vi "RT Driver VI.vi"(6 "Device Clock":string, 9 "Device Inputs FIFO":refnum<k33>, 10 "Device Outputs FIFO":refnum<k33>, 11 "Device Reference":T1 format="%.0x") -> ()   [LabVIEW 2017, in "CD_CI_Test Engine.lvlib"]
uses:
  CD_CI_Test Engine.lvlib
  <vilib>/NI Veristand/Custom Device API/Custom Device Channel Type.ctl
  <vilib>/NI VeriStand/Custom Device API/Custom Device API.lvlib
  <vilib>/NI VeriStand/Custom Device Tools/Custom Device Utility Library/Custom Device Utility Library.lvlib
  <vilib>/NI Veristand/Custom Device API/Custom Device Item Ref.ctl
panel:
  in  "Initialization Status Notifier":refnum<notifier>
  in  "Status Notifier":refnum<notifier>
  # "Custom Device Template\nv1.0"
  # "Use this template as a starting point for creating a custom device code module. The input controls shown here are specially named controls that the system will use to provide the device loop with data. The controls are not required for the device loop to run. For instance, if the device doesn't produce any output data, then you don't need the Device Outputs FIFO control. If you do use these controls, however, they need to have these exact names to be functional."
  # "The optional status notifier element is used to notify the RT engine of the last state of the custom device, and to indicate the device has completed execution. If this control is not used, a default No Error value is returned to the system when the device finishes execution.\n\nNote: This error state is not checked until the system shuts down. Use an output status channel to send more immediate status values to the system."
  # "This optional input can be used to send the VeriStand Engine the final status of the custom device initalization process. If this control exists on the custom device front panel, the VeriStand Engine will wait for a status update before starting up. If the custom device reports an error, that will abort the execution of the current configuration in the VeriStand Engine.\n\nThis control can be deleted if the custom device does not need to send the initialization status update."
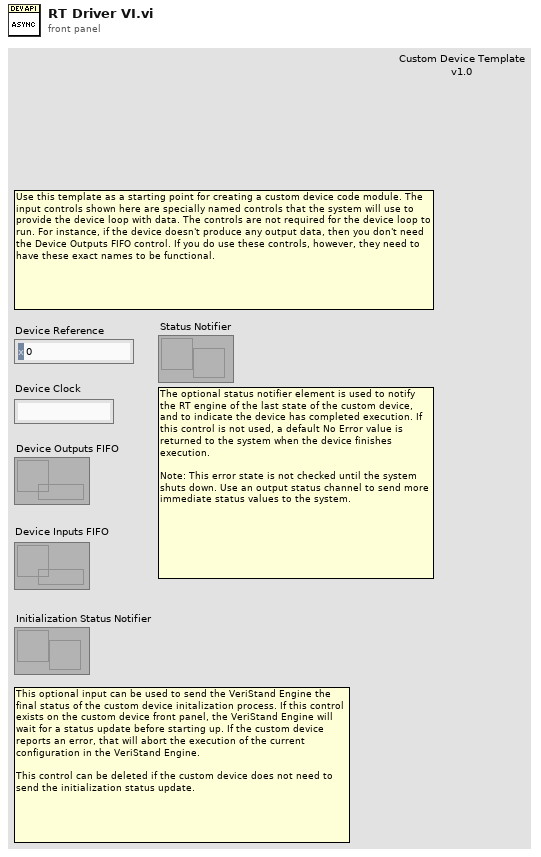
[diagram p1: front panel]
types:
  T1 = typedef "Custom Device API.lvlib/Custom Device Item Ref.ctl" = u64
  T2 = typedef "Custom Device API.lvlib/Custom Device Channel Type.ctl" = enum16{"Input", "Output"}
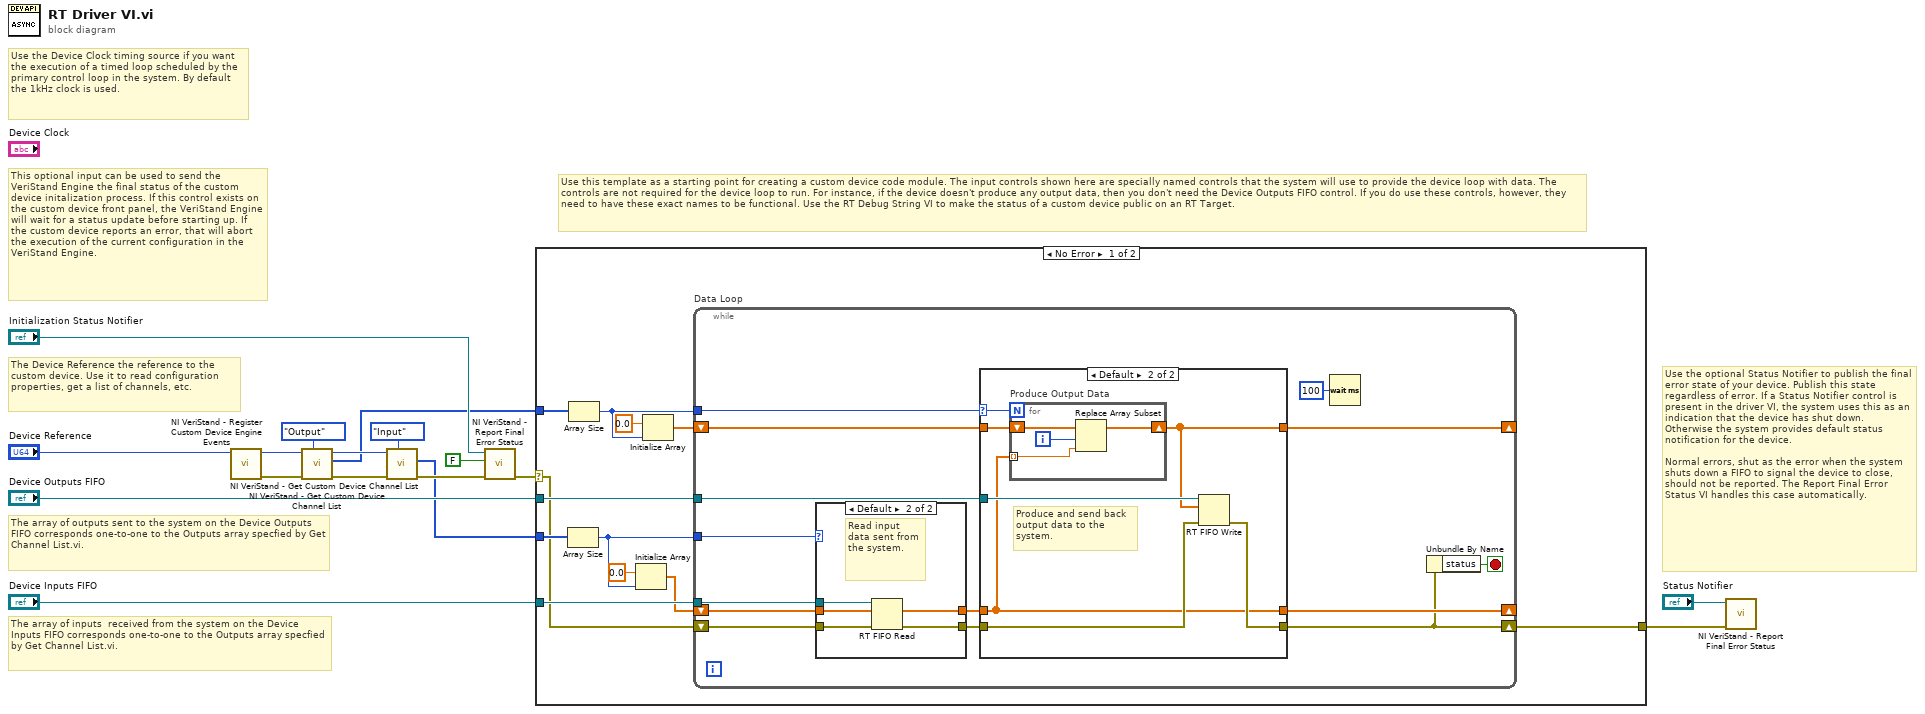
[diagram p0: block diagram]
diagram:
  # "This optional input can be used to send the VeriStand Engine the final status of the custom device initalization process. If this control exists on the custom device front panel, the VeriStand Engine will wait for a status update before starting up. If the custom device reports an error, that will abort the execution of the current configuration in the VeriStand Engine."
  # "The array of inputs  received from the system on the Device Inputs FIFO corresponds one-to-one to the Outputs array specfied by Get Channel List.vi."
  # "Use the optional Status Notifier to publish the final error state of your device. Publish this state regardless of error. If a Status Notifier control is present in the driver VI, the system uses this as an indication that the device has shut down. Otherwise the system provides default status notification for the device.\n\nNormal errors, shut as the error when the system shuts down a FIFO to signal the device to close, should not be reported. The Report Final Error Status VI handles this case automatically."
  # "The array of outputs sent to the system on the Device Outputs FIFO corresponds one-to-one to the Outputs array specfied by Get Channel List.vi."
  # "The Device Reference the reference to the custom device. Use it to read configuration properties, get a list of channels, etc."
  # "Use the Device Clock timing source if you want the execution of a timed loop scheduled by the primary control loop in the system. By default the 1kHz clock is used."
  # "Use this template as a starting point for creating a custom device code module. The input controls shown here are specially named controls that the system will use to provide the device loop with data. The controls are not required for the device loop to run. For instance, if the device doesn't produce any output data, then you don't need the Device Outputs FIFO control. If you do use these controls, however, they need to have these exact names to be functional. Use the RT Debug String VI to make the status of a custom device public on an RT Target."
  n1 = call <vilib>:"NI VeriStand - Register Custom Device Engine Events.vi"("Device Ref in"="Device Reference") -> ("error out"=w17:errorcluster, "Device Ref out"=w3:T1)  [unwired: 8 in, 1 out]
  n2 = call <vilib>:"NI VeriStand - Get Custom Device Channel List.vi"("Channel Type"=Custom_Device_Channel_Type."Output", "error in (no error)"=w17, "Device Ref in"=w3) -> ("error out"=w10:errorcluster, "Specified Channel Ref List"=w7:T1[], "Device Ref out"=w11:T1)  [unwired: 6 out]
  n3 = call <vilib>:"NI VeriStand - Get Custom Device Channel List.vi"("Channel Type"=Custom_Device_Channel_Type."Input", "error in (no error)"=w10, "Device Ref in"=w11) -> ("error out"=w16:errorcluster, "Specified Channel Ref List"=w8:T1[])  [unwired: 7 out]
  n4 = call <vilib>:"NI VeriStand - Report Final Error Status.vi"("error in (no error)"=w16, "Filter FIFO & Shutdown Errors (T)"=FALSE ("Filter FIFO Errors (T)"), "Status Notifier"="Initialization Status Notifier") -> ("error out"=w2:errorcluster)  [unwired: 8 out]
  n5 = case shown="No Error" w2 {
    selector: w2 -> [w18 w65]
    tunnel: "Device Outputs FIFO" -> [w29 _]
    tunnel: "Device Inputs FIFO" -> [w28 _]
    tunnel: w8 -> [w22 _]
    tunnel: w7 -> [w21 _]
    tunnel: [w19 w65] -> w5
    frame No Error {
      n6 = Array Size(array=w22) -> (size(s)=w20:i32)
      n7 = Array Size(array=w21) -> (size(s)=w23:i32)
      n8 = Initialize Array(0.0 ("element"), w20) -> (w24:dbl[])
      n9 = Initialize Array(0.0 ("element"), w23) -> (w25:dbl[])
      n10 = while "Data Loop" {
        shift-right: [w41] -> _
        shift-left: w24 -> [w42]
        shift-right: [w34] -> w19
        shift-left: w18 -> [w43]
        shift-right: [w39] -> _
        shift-left: w25 -> [w40]
        tunnel: w23 -> [w36]
        tunnel: w29 -> [w38]
        tunnel: w28 -> [w37]
        tunnel: w20 -> [w35]
        stop <- w33 stop-if-true
        n11 = case shown="Default" w35 {
          tunnel: w37 -> [_ w64]
          tunnel: w42 -> [w59 w63]
          tunnel: [w59 w62] -> w32
          tunnel: [w58 w61] -> w31
          tunnel: w43 -> [w58 w60]
          frame 0 {
            # "No inputs to read\nfrom system. Inputs FIFO not created in this case, so don't write to it."
          }
          frame Default {
            # "Read input data sent from the system."
            n12 = RT FIFO Read(0:w64, 1:w63, 3:w60) -> (9:w62:dbl[], 11:w61:errorcluster)  [unwired: 4 out]
          }
        }
        n13 = case shown="Default" w36 {
          selector: w36 -> [_ w48]
          tunnel: w38 -> [_ w53]
          tunnel: w40 -> [w46 w52]
          tunnel: w32 -> [w45 w49]
          tunnel: w31 -> [w44 w51]
          tunnel: [w44 w50] -> w34
          tunnel: [w46 w47] -> w39
          tunnel: [w45 w49] -> w41
          frame 0 {
            # "No outputs to write to system. The Device Outputs FIFO is never created in this case, so don't write to it."
          }
          frame Default {
            # "Produce and send back output data to the system."
            n14 = for "Produce Output Data" {
              N: w48 -> [_]
              shift-right: [w56] -> w47
              shift-left: w52 -> [w57]
              tunnel: w49 -> [w54] mode=indexing
              i -> [w55]
              n15 = Replace Array Subset(array=w57, new element=w54, index=w55) -> (w56:dbl[])
            }
            n16 = RT FIFO Write(0:w53, 1:w47, 3:w51) -> (11:w50:errorcluster)  [unwired: 1 in, 4 out]
          }
        }
        n17 = Wait (ms)(milliseconds to wait=u32 100) -> ()  [unwired: 1 out]
        n18 = Unbundle By Name(w34) -> ("status"=w33:bool)
      }
    }
    frame Error {
    }
  }
  n19 = call <vilib>:"NI VeriStand - Report Final Error Status.vi"("error in (no error)"=w5, "Status Notifier"="Status Notifier") -> ()  [unwired: 1 in, 9 out]
